vi "Jeff stuff.vi"() -> ()   [LabVIEW 2018]
uses:
  <vilib>/Rock Robotics/SystemInterfaces/AI/FPGA_AIGyroChannel.ctl
  <vilib>/Rock Robotics/WPI/Gyro/WPI_GyroAnalogOpen.vi
panel:
  out "Epic":dbl(slide) scale=0.0..10.0
  in  "Motor":dbl(slide) scale=0.0..10.0
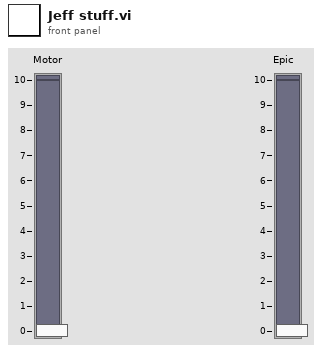
[diagram p1: front panel]
types:
  T1 = typedef "FPGA_AIGyroChannel.ctl" = enum8{"AI 0", "AI 1", "Invalid"}
  T2 = typedef "WPI_GyroDevRef.ctl" = cluster{"DevStatus":errorcluster, "Analog Channel":T3, "Gain (VoltsPerDegree/Second)":dbl, "Gyro Type":enum16{"Analog", "XRS450"}, "Handle":i32, "SPI Bus":T4, "Device Found":bool, "Sample Rate":dbl, "Calibrate On Open":bool, "Offset":dbl}
  T3 = typedef "FPGA_AIChannel.ctl" = enum8{"AI 0", "AI 1", "AI 2", "AI 3", "AI MXP 0", "AI MXP 1", "AI MXP 2", "AI MXP 3", "Invalid"}
  T4 = typedef "spi_bus.ctl" = enum16{"SPI On-Board, CS0", "SPI On-Board, CS1", "SPI On-Board, CS2", "SPI On-Board, CS3", "SPI MXP", "Invalid"}
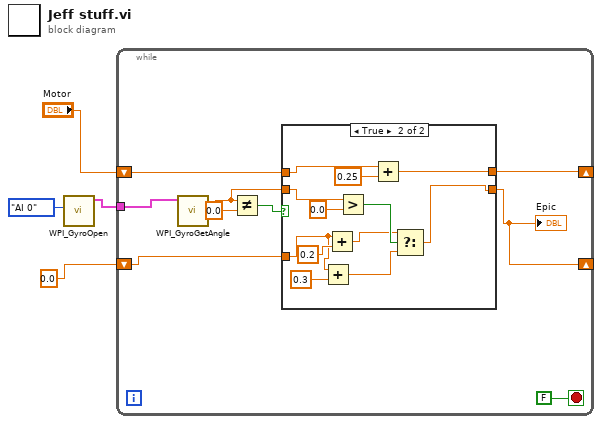
[diagram p0: block diagram]
diagram:
  n1 = call-poly <vilib>:"WPI_GyroOpen.vi"("Analog Channel"=FPGA_AIGyroChannel."AI 0") -> ("GyroDevRef"=w3:T2)  [unwired: 8 in, 2 out]
  n2 = while {
    tunnel: w3 -> [w12]
    shift-right: [w7] -> _
    shift-left: "Motor" -> [w8]
    shift-right: [w5] -> _
    shift-left: 0.0 -> [w6]
    stop <- FALSE stop-if-true
    n3 = call <vilib>:"WPI_GyroGetAngle.vi"("GyroDevRef"=w12) -> ("Angle"=w9:dbl)  [unwired: 7 in, 3 out]
    n4 = Not Equal?(x=w9, y=0.0) -> (x != y?=w10:bool)
    n5 = case shown="True" w10 {
      tunnel: w8 -> [w15 w24]
      tunnel: [w14 w16] -> w5
      tunnel: w9 -> [_ w27]
      tunnel: [w15 w22] -> w7
      tunnel: w6 -> [w14 w18]
      frame False {
      }
      frame True {
        n6 = Add(x=w18, y=0.3) -> (x+y=w17:dbl)
        n7 = Add(x=w18, y=0.2) -> (x+y=w20:dbl)
        n8 = Greater?(x=w27, y=0.0) -> (0:w25:bool)
        n9 = Add(x=w24, y=0.25) -> (x+y=w22:dbl)
        n10 = Select(t=w20, s=w25, f=w17) -> (s? t:f=w16:dbl)
      }
    }
    "Epic" <- w5
  }
